vi "DynamicSubtractU8Baseline.vi"(8 "Last? Input":bool, 9 "Baseline U8":u8, 11 "IO Module\\Synchronous Trigger Input":u8) -> (0 "Last? Output":bool, 2 "Trigger Edge Array":bool[](array[boolean]), 3 "Baseline Array Output":u8[](array[numeric]))   [LabVIEW 2012]
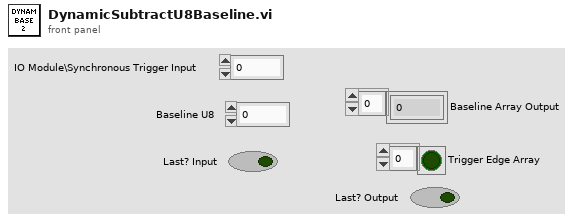
[diagram p1: front panel]
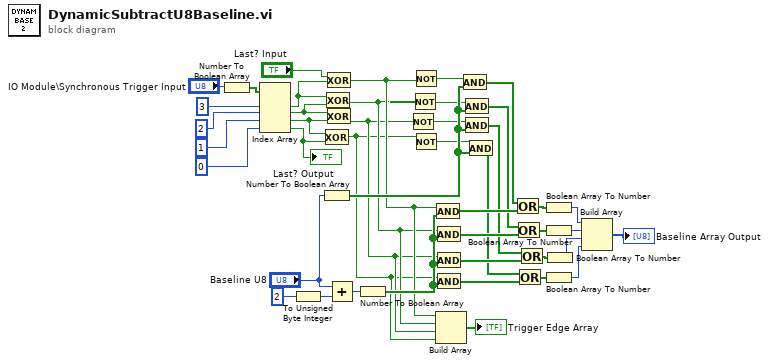
[diagram p0: block diagram]
diagram:
  n1 = Number To Boolean Array(number="IO Module\\Synchronous Trigger Input") -> (Boolean array=w43:bool[])
  n2 = Index Array(array=w43, index #1=3 ("index"), index #2=2 ("index"), index #3=1 ("index"), index #4=0 ("index")) -> (element #1=w34:bool, element #2=w33:bool, element #3=w32:bool, element #4=w31:bool)
  "Last? Output" <- w31
  n3 = To Unsigned Byte Integer(number=i16 2) -> (unsigned 8bit integer=w36:u8)
  n4 = Exclusive Or(1:w31, 2:w32) -> (0:w2:bool)
  n5 = Number To Boolean Array(number="Baseline U8") -> (Boolean array=w30:bool[])
  n6 = Exclusive Or(1:w33, 2:w34) -> (0:w4:bool)
  n7 = Exclusive Or(1:w34, 2:"Last? Input") -> (0:w5:bool)
  n8 = Exclusive Or(1:w32, 2:w33) -> (0:w3:bool)
  n9 = Add(x="Baseline U8", y=w36) -> (x+y=w6:u8)
  n10 = Number To Boolean Array(number=w6) -> (Boolean array=w29:bool[])
  n11 = Not(x=w3) -> (.not. x?=w22:bool)
  n12 = Not(x=w4) -> (.not. x?=w23:bool)
  n13 = Not(x=w5) -> (.not. x?=w24:bool)
  n14 = Not(x=w2) -> (.not. x?=w21:bool)
  n15 = And(x=w5, y=w29) -> (x .and. y?=w12:bool[])
  n16 = And(x=w4, y=w29) -> (x .and. y?=w13:bool[])
  n17 = And(x=w3, y=w29) -> (x .and. y?=w14:bool[])
  n18 = And(x=w2, y=w29) -> (x .and. y?=w15:bool[])
  n19 = Build Array(w5, w4, w3, w2) -> (→"Trigger Edge Array":bool[])
  n20 = And(x=w24, y=w30) -> (x .and. y?=w11:bool[])
  n21 = And(x=w23, y=w30) -> (x .and. y?=w10:bool[])
  n22 = And(x=w22, y=w30) -> (x .and. y?=w9:bool[])
  n23 = And(x=w21, y=w30) -> (x .and. y?=w8:bool[])
  n24 = Or(x=w11, y=w12) -> (x .or. y?=w19:bool[])
  n25 = Or(x=w10, y=w13) -> (x .or. y?=w16:bool[])
  n26 = Or(x=w8, y=w15) -> (x .or. y?=w18:bool[])
  n27 = Or(x=w9, y=w14) -> (x .or. y?=w17:bool[])
  n28 = Boolean Array To Number(Boolean array=w19) -> (number=w28:u8)
  n29 = Boolean Array To Number(Boolean array=w16) -> (number=w27:u8)
  n30 = Boolean Array To Number(Boolean array=w18) -> (number=w25:u8)
  n31 = Boolean Array To Number(Boolean array=w17) -> (number=w26:u8)
  n32 = Build Array(w28, w27, w26, w25) -> (→"Baseline Array Output":u8[])
